vi "HMI.vi"() -> ()   [LabVIEW 2019, in "HMI Class 3.lvclass"]
uses:
  HMI Class 3.lvclass
  Class 2.lvclass
  Datos Out.vi
  Datos In.vi
panel:
  in  "MODO PRODUCCION":bool
  out "mensajes a usuario":string
  in  "PARO DE E":bool
  in  "Test":bool
  out "Numeric":dbl
  in  "MODO MANUAL":bool
  in  "stop":bool
  in  "INICIO":bool
  out "FALLA PRESENTE":bool
  out "MAQUINA EN ORIGEN":bool
  in  "RESET":bool
  in  "Tab Control":enum32{"0", "1", "2", "3", "4"}(tab)
  in  "MOVER A ORIGEN":bool
  in  "Nombre":string
  in  "Clave":string
  in  "ENTER":bool
  out "?":string
  out "PIEZAS YIELD":string
  out "PIEZAS MALAS":string
  out "LOTE ACTUAL":string
  out "JOB":string
  out "MODELO":string
  out "PIEZA 2":bool
  out "PIEZA":bool
  out "LIMITE MINIMO":dbl min=0.0 max=9999.0
  out "LIMITE MAXIMO":dbl min=0.0 max=9999.0
  out "LIMITE MINIMO":dbl min=0.0 max=9999.0
  out "LIMITE MAXIMO":dbl min=0.0 max=9999.0
  out "ESTADO DE PIEZA TENSION":string
  out "ESTADO DE PIEZA GAP":string
  out "VALOR DE DISTANCIA":dbl
  out "SIN CAMBIOS":bool
  out "PIEZAS BUENAS":string
  out "CON CAMBIOS":bool
  out "VALOR DE TENSIÓN":dbl
  out "SMAC SEGURO":bool
  out "PIEZA EN NIDO":bool
  in  "MANUAL":bool
  out "SMAC MUESTRA":bool
  out "SMAC APROX":bool
  in  "SMAC AVANZANDO":bool
  in  "SMAC RETORNANDO":bool
  in  "CILINDRO 2":bool
  in  "CILINDRO 1":bool
  out "SMAC AV. SEGURO":bool
  out "SMAC HOME":bool
  out "BIMANUAL 2":bool
  out "BIMANUAL 1":bool
  out "AVANCE CILINDRO 2":bool
  out "HOME CILINDRO 2":bool
  out "AVANCE CILINDRO 1":bool
  out "HOME CILINDRO 1":bool
  out "PIEZA":bool
  in  "LIMITE MINIMO":dbl min=0.0 max=9999.0
  in  "LIMITE MAXIMO 4":dbl min=0.0 max=9999.0
  out "ESTADO DE PIEZA GAP":string
  out "VALOR DE DISTANCIA":dbl
  in  "EST 2":bool
  out "PIEZA":bool
  in  "LIMITE MINIMO":dbl min=0.0 max=9999.0
  in  "LIMITE MAXIMO":dbl min=0.0 max=9999.0
  out "ESTADO DE PIEZA TENSION":string
  out "VALOR DE TENSIÓN":dbl
  in  "EST 1":bool
  out "SIN CAMBIOS":bool
  out "CON CAMBIOS":bool
  in  "EST 3":bool
  in  "MODO INGENIERIA":bool
  in  "MODO DE OPERACION":bool
  # "MENÚ PRINCIPAL"
  # "MODO DE OPERACIÓN"
  # "ESTACION 1\n PRUEBA TENSIÓN"
  # "ESTACION 2\n PRUEBA GAP"
  # "ESTACION 3\n PRUEBA TRIP-GAP"
  # "CONTINUAIDAD EN CONTACTOS"
  # "PRODUCCIÓN"
  # "SENSORES"
  # "CILINDROS"
  # "SEGURIDAD"
  # "ESTADO DEL SMAC"
  # "SMAC"
  # "ENTRADAS   MODO MANUAL    SALIDAS"
  # "SELECCION MODELO \nDE PIEZA"
  # "AGREGAR MODELO"
  # "ESTACION 1\n PRUEBA TENSIÓN"
  # "ESTACION 2\n PRUEBA GAP"
  # "ESTACION 3\n PRUEBA TRIP-GAP"
  # "CONTINUAIDAD EN CONTACTOS"
  # "MODO INGENIERIA\nCONFIGURACION DE PARAMETROS"
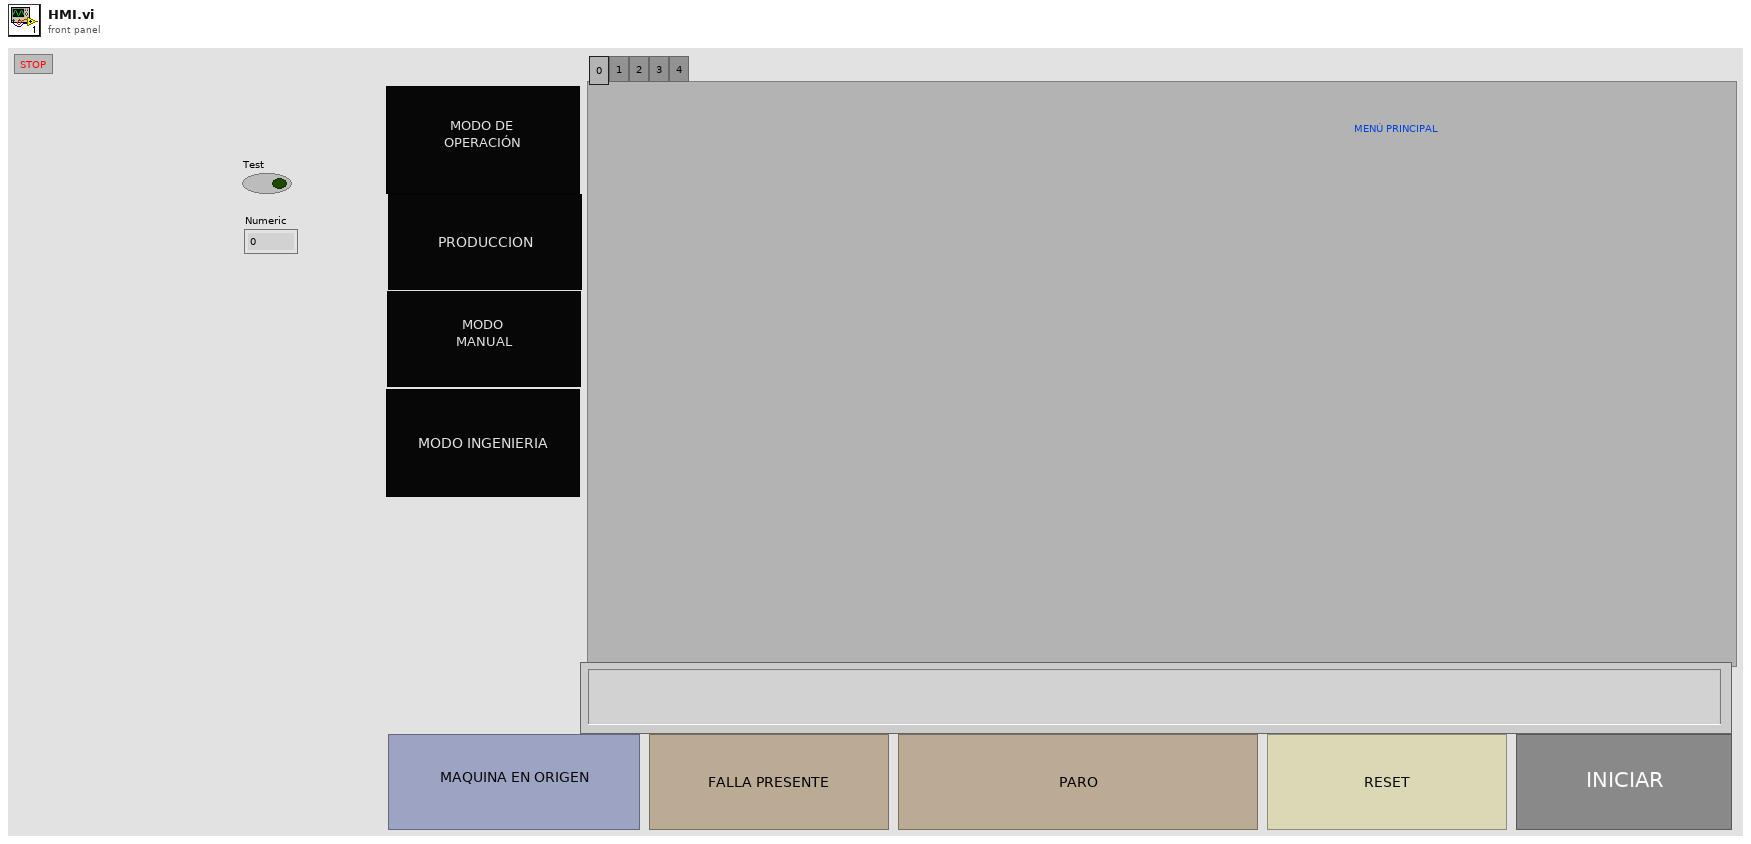
[diagram p1: front panel]
types:
  T1 = enum8{"Enabled", "Disabled", "Disabled and Grayed Out"}
  T2 = cluster{"Test":bool, "CILINDRO _1":bool, "CILINDRO _2":bool, "SMAC_RETORNANDO":bool, "SMAC_AVANZANDO":bool, "MANUAL":bool, "EST_1":bool, "EST_2":bool, "EST_3":bool, "MOVER A ORIGEN":bool, "RESET":bool, "PARO":bool, "INICIO":bool, "DATA_CONTROL":cluster{"ESTACION_1":cluster{"ACEPTADA":bool, "MAXIMO":dbl, "MINIMO":dbl, "LECTURA":dbl}, "ESTACION_2":cluster{"ACEPTADA":bool, "MAXIMO":dbl, "MINIMO":dbl, "LECTURA":dbl}, "ESTACION_3":cluster{"ACEPTADA":bool, "MAXIMO":dbl, "MINIMO":dbl, "LECTURA":dbl}}, "INGENIERIA O PROCESO":bool}
  T3 = cluster{"SALIDAS.CILINDRO 1":bool, "SALIDAS.CILINDRO 2":bool, "SALIDAS.SEMAC RETORNANDO":bool, "SALIDAS.SAMAC AVANZANDO":bool, "Auto(off)/Manual(on)":bool, "HOME_CILINDRO_1":bool, "HOME_CILINDRO_2":bool, "AVANCE_CILINDRO_1":bool, "AVANCE_CILINDRO_2":bool, "PIEZA_EN_NIDO":bool, "BIMANUAL 2":bool, "BIMANUAL1":bool, "SIN CAMBIOS":bool, "CON  CAMBIOS":bool, "TESTER":bool, "MAQUINA EN ORIGEN":bool, "FALLA PRESENTE":bool}
  T4 = cluster{"Numeric":dbl, "VALOR DE DISTANCIA":dbl, "VALOR DE TENSION":dbl}
  T5 = cluster{"DATO GAP":string, "DATO TENSION":string, "mensajes usuario":string}
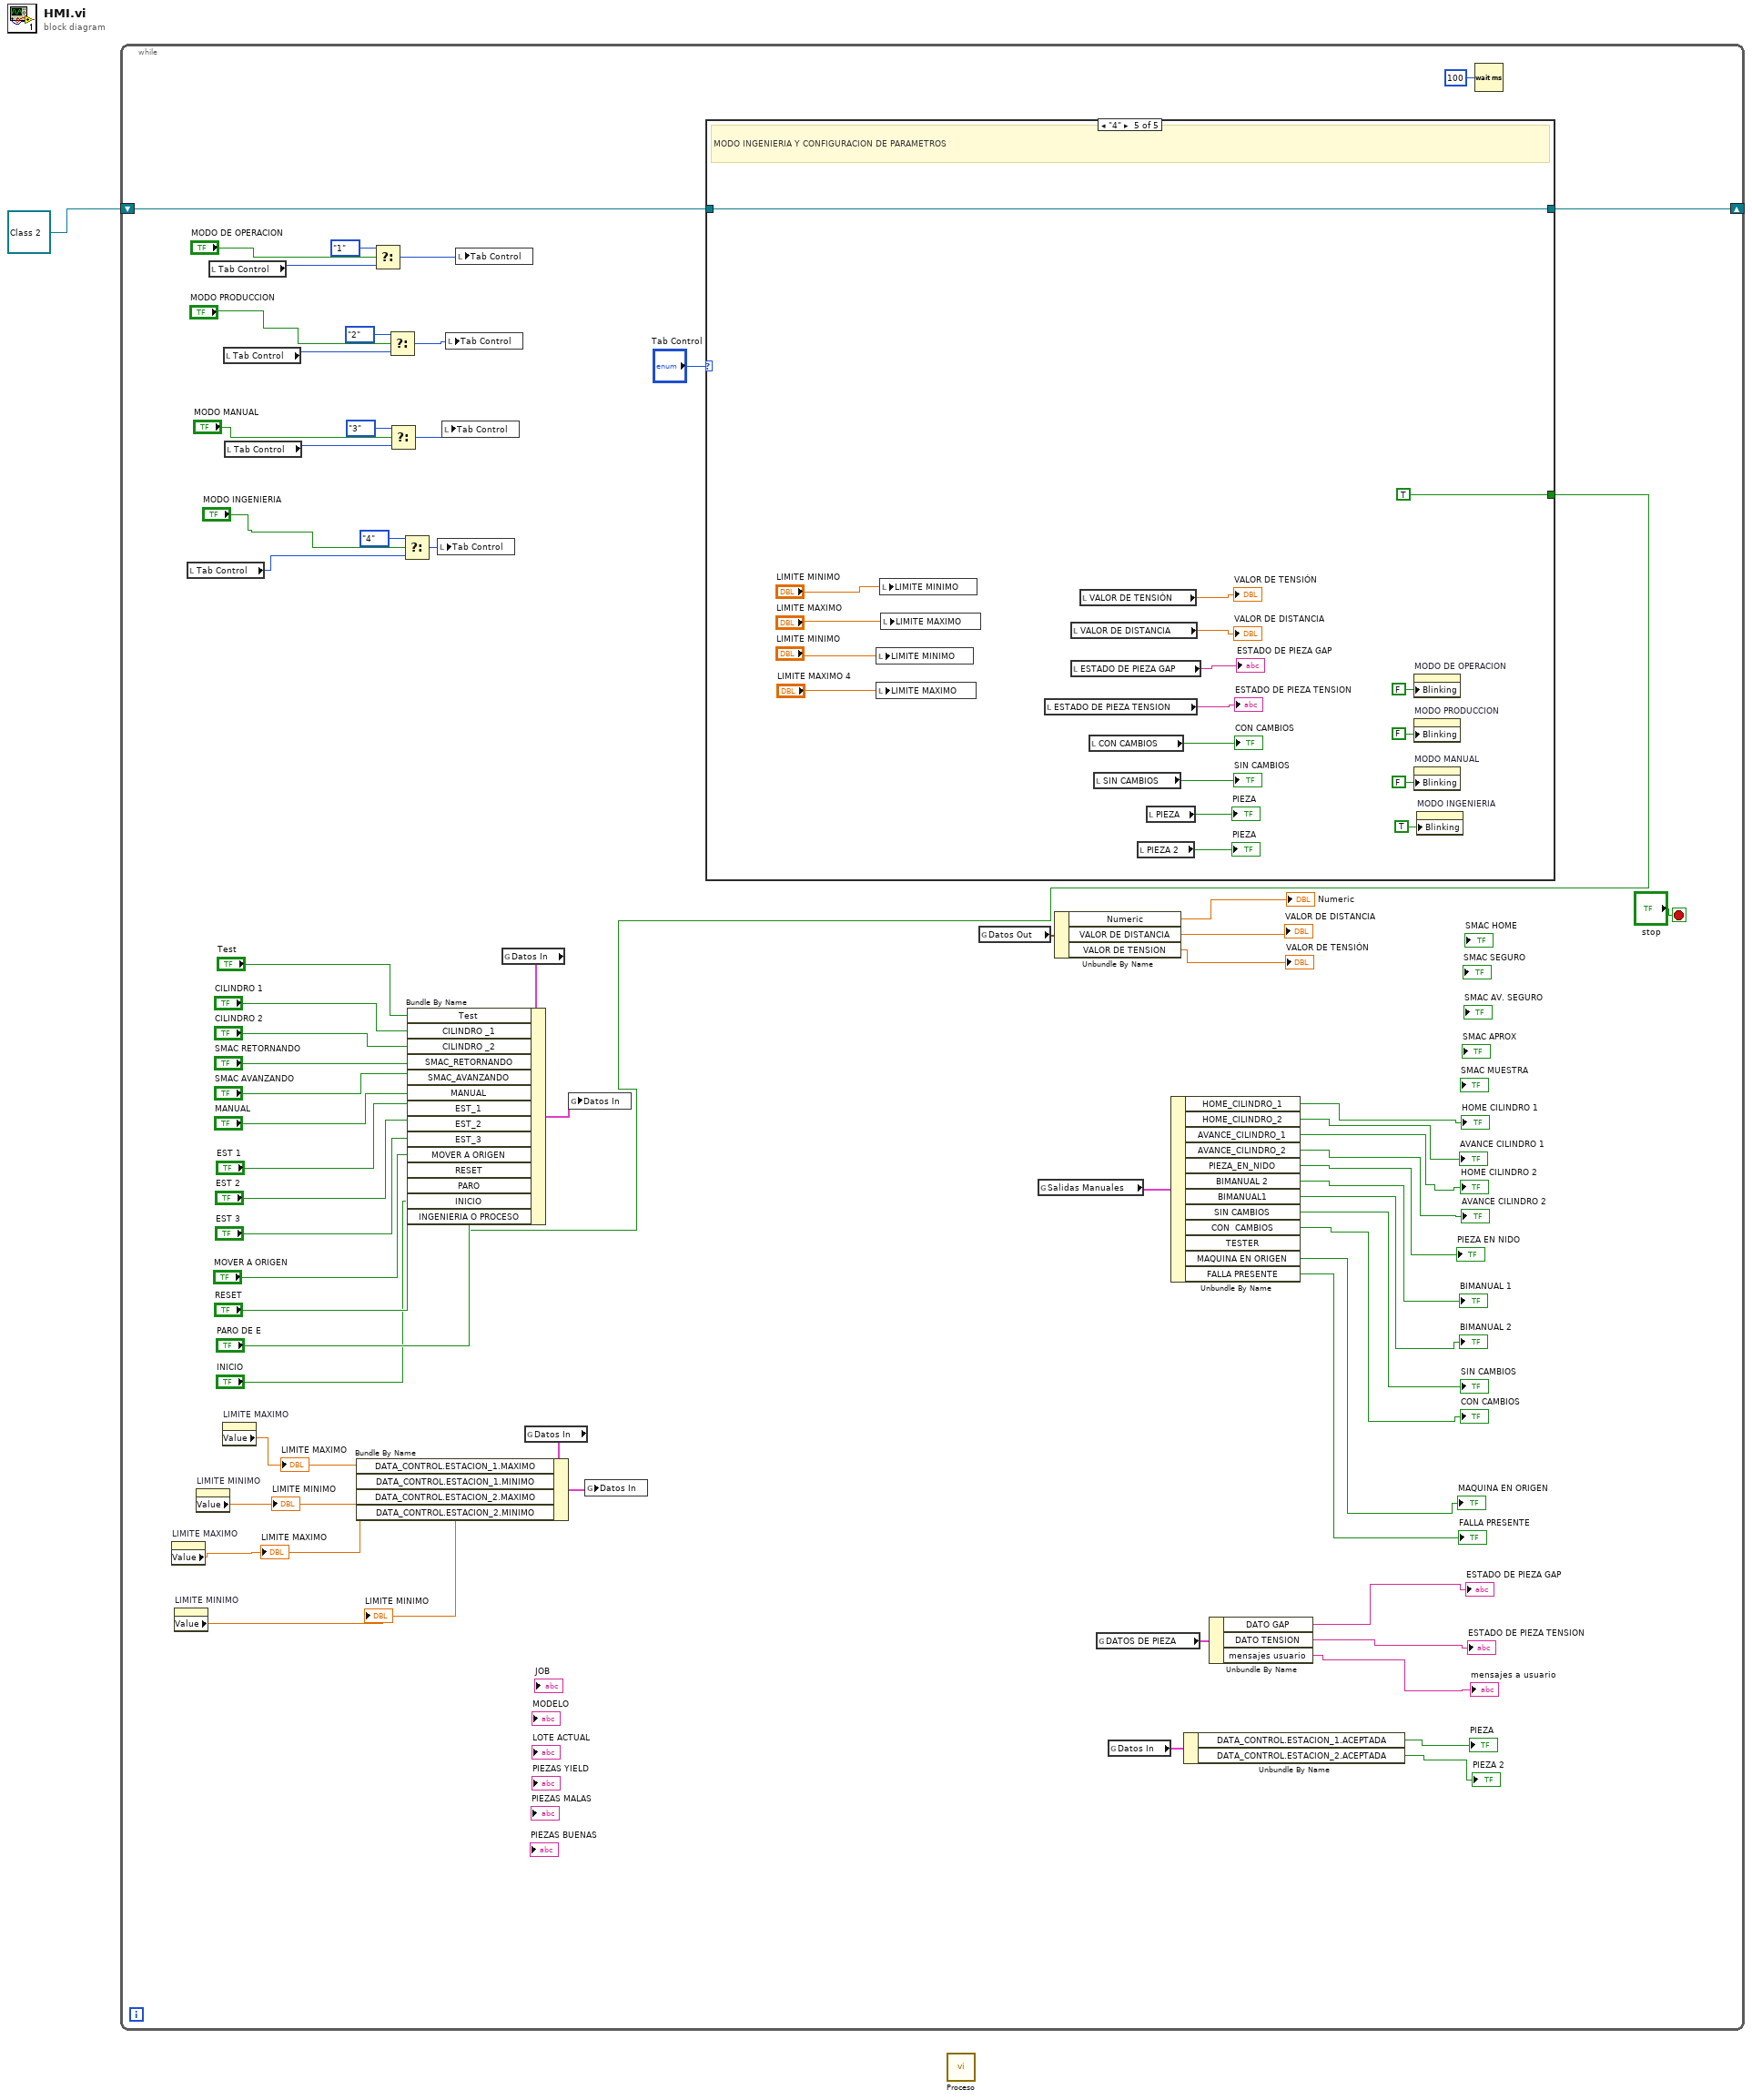
[diagram p0: block diagram]
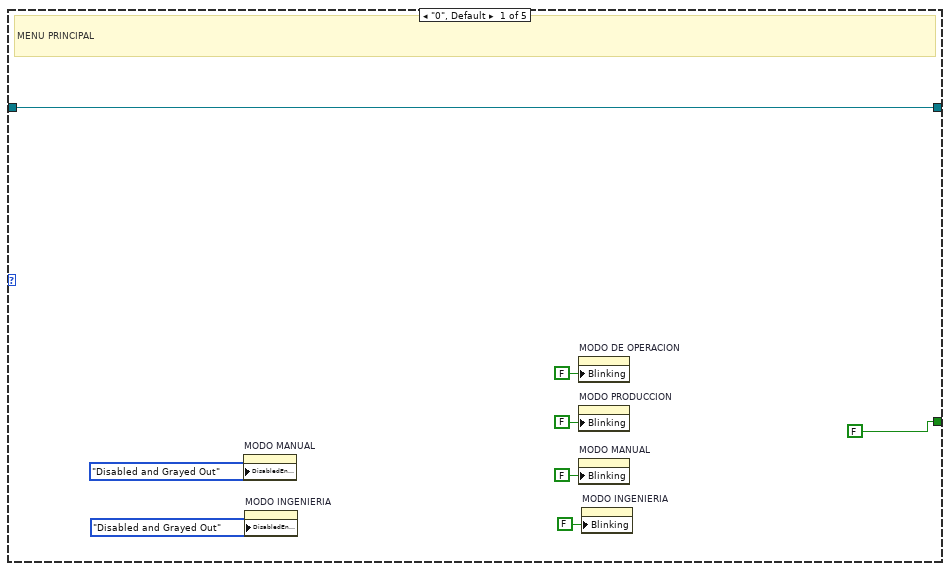
[diagram p2: hidden frame]
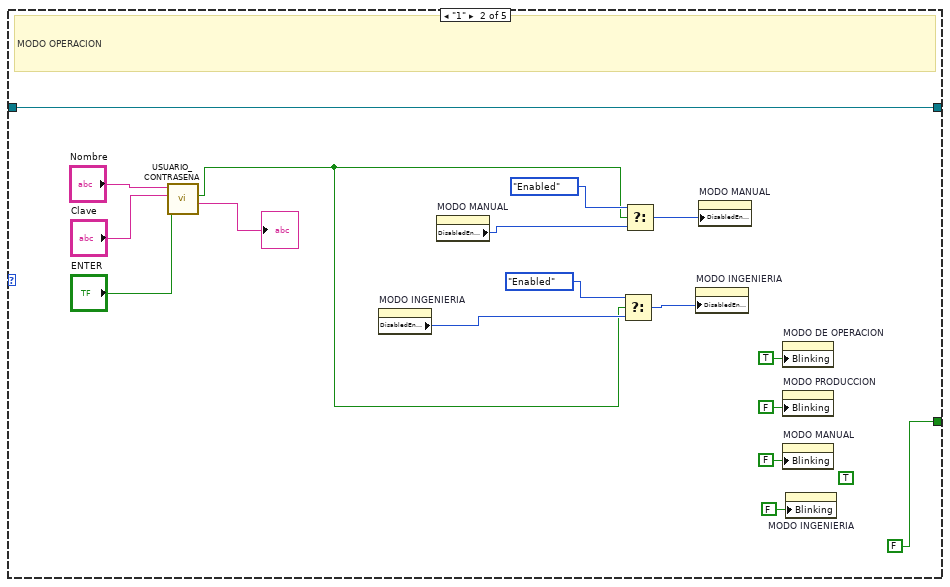
[diagram p3: hidden frame]
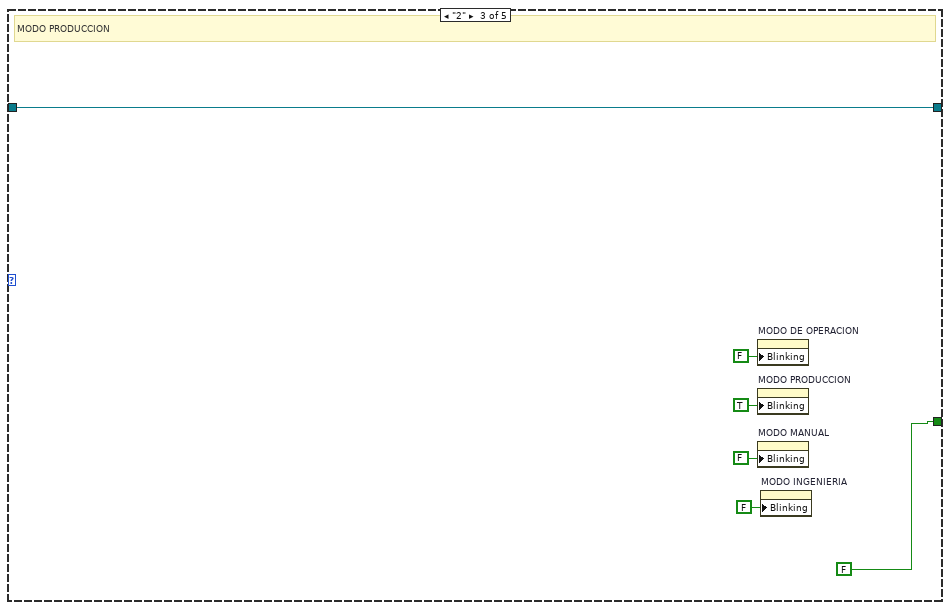
[diagram p4: hidden frame]
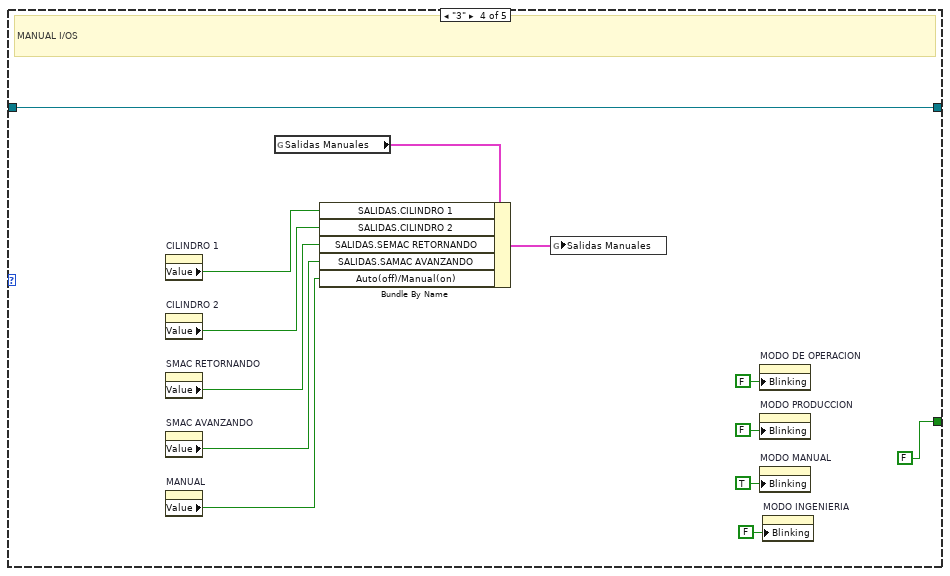
[diagram p5: hidden frame]
diagram:
  n1 = while {
    shift-right: [w64] -> _
    shift-left: refnum<class "Class 2.lvclass"> refnum ("Class 2.lvclass") -> [w65]
    stop <- "stop" stop-if-true
    n2 = property on="LIMITE MAXIMO" class="DigNum (strict)"() -> ("Value"=w4:dbl)  [unwired: 2 in, 2 out]
    "LIMITE MAXIMO" <- w4
    n3 = property on="LIMITE MINIMO" class="DigNum (strict)"() -> ("Value"=w5:dbl)  [unwired: 2 in, 2 out]
    "LIMITE MINIMO" <- w5
    n4 = local read "Tab Control"() -> (w19:enum32{"0", "1", "2", "3", "4"})
    n5 = property on="LIMITE MINIMO" class="DigNum (strict)"() -> ("Value"=w6:dbl)  [unwired: 2 in, 2 out]
    "LIMITE MINIMO" <- w6
    n6 = local read "Tab Control"() -> (w59:enum32{"0", "1", "2", "3", "4"})
    n7 = property on="LIMITE MAXIMO" class="DigNum (strict)"() -> ("Value"=w7:dbl)  [unwired: 2 in, 2 out]
    "LIMITE MAXIMO" <- w7
    n8 = local read "Tab Control"() -> (w11:enum32{"0", "1", "2", "3", "4"})
    n9 = local read "Tab Control"() -> (w15:enum32{"0", "1", "2", "3", "4"})
    n10 = Select(t=enum32{"0", "1", "2", "3", "4", "5", "6", "7"}."1", s="MODO DE OPERACION", f=w59) -> (s? t:f=w57:enum32{"0", "1", "2", "3", "4", "5", "6", "7"})
    n11 = Select(t=enum32{"0", "1", "2", "3", "4", "5", "6", "7"}."2", s="MODO PRODUCCION", f=w11) -> (s? t:f=w10:enum32{"0", "1", "2", "3", "4", "5", "6", "7"})
    n12 = Select(t=enum32{"0", "1", "2", "3", "4", "5", "6", "7"}."3", s="MODO MANUAL", f=w15) -> (s? t:f=w13:enum32{"0", "1", "2", "3", "4", "5", "6", "7"})
    n13 = Select(t=enum32{"0", "1", "2", "3", "4", "5", "6", "7"}."4", s="MODO INGENIERIA", f=w19) -> (s? t:f=w17:enum32{"0", "1", "2", "3", "4", "5", "6", "7"})
    n14 = local write "Tab Control"(w17) -> ()
    n15 = local write "Tab Control"(w13) -> ()
    n16 = local write "Tab Control"(w10) -> ()
    n17 = local write "Tab Control"(w57) -> ()
    n18 = global read "Datos In.vi" "Datos In"() -> (w31:T2)
    n19 = global read "Datos In.vi" "Datos In"() -> (w24:T2)
    n20 = Bundle By Name(cluster=w24, "DATA_CONTROL.ESTACION_1.MAXIMO"=w7, "DATA_CONTROL.ESTACION_1.MINIMO"=w6, "DATA_CONTROL.ESTACION_2.MAXIMO"=w4, "DATA_CONTROL.ESTACION_2.MINIMO"=w5) -> (w23:T2)
    n21 = global write "Datos In.vi" "Datos In"(w23) -> ()
    n22 = case shown="\"4\"" "Tab Control" {
      tunnel: w65 -> [w75 w92 w98 w111 w129]
      tunnel: [w75 w92 w98 w111 w129] -> w64
      tunnel: [FALSE FALSE FALSE FALSE TRUE] -> w2
      frame "0", Default {
        # "MENU PRINCIPAL"
        n23 = property on="MODO MANUAL" class="Bool (strict)"("DisabledEnum"=T1."Disabled and Grayed Out" ("Disabled")) -> ()  [unwired: 2 in, 2 out]
        n24 = property on="MODO INGENIERIA" class="Bool (strict)"("DisabledEnum"=T1."Disabled and Grayed Out" ("Disabled")) -> ()  [unwired: 2 in, 2 out]
        n25 = property on="MODO DE OPERACION" class="Bool (strict)"("Blinking"=FALSE) -> ()  [unwired: 2 in, 2 out]
        n26 = property on="MODO PRODUCCION" class="Bool (strict)"("Blinking"=FALSE) -> ()  [unwired: 2 in, 2 out]
        n27 = property on="MODO MANUAL" class="Bool (strict)"("Blinking"=FALSE) -> ()  [unwired: 2 in, 2 out]
        n28 = property on="MODO INGENIERIA" class="Bool (strict)"("Blinking"=FALSE) -> ()  [unwired: 2 in, 2 out]
      }
      frame "1" {
        (unwired) TRUE
        # "MODO OPERACION"
        n29 = call "USUARIO_CONTRASENA.vi"("INGRESAR (ENTER)"="ENTER", "Clave"="Clave", "Nombre"="Nombre") -> ("String 2"=→"?":string, "ACCESO"=w77:bool)  [unwired: 7 in]
        n30 = property on="MODO INGENIERIA" class="Bool (strict)"() -> ("DisabledEnum"=w86:T1)  [unwired: 2 in, 2 out]
        n31 = property on="MODO MANUAL" class="Bool (strict)"() -> ("DisabledEnum"=w87:T1)  [unwired: 2 in, 2 out]
        n32 = Select(t=T1."Enabled" ("Disabled"), s=w77, f=w86) -> (s? t:f=w90:T1)
        n33 = Select(t=T1."Enabled" ("Disabled"), s=w77, f=w87) -> (s? t:f=w91:T1)
        n34 = property on="MODO INGENIERIA" class="Bool (strict)"("DisabledEnum"=w90) -> ()  [unwired: 2 in, 2 out]
        n35 = property on="MODO MANUAL" class="Bool (strict)"("DisabledEnum"=w91) -> ()  [unwired: 2 in, 2 out]
        n36 = property on="MODO DE OPERACION" class="Bool (strict)"("Blinking"=TRUE) -> ()  [unwired: 2 in, 2 out]
        n37 = property on="MODO PRODUCCION" class="Bool (strict)"("Blinking"=FALSE) -> ()  [unwired: 2 in, 2 out]
        n38 = property on="MODO MANUAL" class="Bool (strict)"("Blinking"=FALSE) -> ()  [unwired: 2 in, 2 out]
        n39 = property on="MODO INGENIERIA" class="Bool (strict)"("Blinking"=FALSE) -> ()  [unwired: 2 in, 2 out]
      }
      frame "2" {
        # "MODO PRODUCCION"
        n40 = property on="MODO DE OPERACION" class="Bool (strict)"("Blinking"=FALSE) -> ()  [unwired: 2 in, 2 out]
        n41 = property on="MODO PRODUCCION" class="Bool (strict)"("Blinking"=TRUE) -> ()  [unwired: 2 in, 2 out]
        n42 = property on="MODO MANUAL" class="Bool (strict)"("Blinking"=FALSE) -> ()  [unwired: 2 in, 2 out]
        n43 = property on="MODO INGENIERIA" class="Bool (strict)"("Blinking"=FALSE) -> ()  [unwired: 2 in, 2 out]
      }
      frame "3" {
        # "MANUAL I/OS"
        n44 = property on="CILINDRO 1" class="Bool (strict)"() -> ("Value"=w110:bool)  [unwired: 2 in, 2 out]
        n45 = property on="CILINDRO 2" class="Bool (strict)"() -> ("Value"=w109:bool)  [unwired: 2 in, 2 out]
        n46 = property on="SMAC RETORNANDO" class="Bool (strict)"() -> ("Value"=w108:bool)  [unwired: 2 in, 2 out]
        n47 = property on="SMAC AVANZANDO" class="Bool (strict)"() -> ("Value"=w107:bool)  [unwired: 2 in, 2 out]
        n48 = property on="MANUAL" class="Bool (strict)"() -> ("Value"=w106:bool)  [unwired: 2 in, 2 out]
        n49 = global read "Datos Out.vi" "Salidas Manuales"() -> (w105:T3)
        n50 = Bundle By Name(cluster=w105, "SALIDAS.CILINDRO 1"=w110, "SALIDAS.CILINDRO 2"=w109, "SALIDAS.SEMAC RETORNANDO"=w108, "SALIDAS.SAMAC AVANZANDO"=w107, "Auto(off)/Manual(on)"=w106) -> (w104:T3)
        n51 = global write "Datos Out.vi" "Salidas Manuales"(w104) -> ()
        n52 = property on="MODO DE OPERACION" class="Bool (strict)"("Blinking"=FALSE) -> ()  [unwired: 2 in, 2 out]
        n53 = property on="MODO PRODUCCION" class="Bool (strict)"("Blinking"=FALSE) -> ()  [unwired: 2 in, 2 out]
        n54 = property on="MODO MANUAL" class="Bool (strict)"("Blinking"=TRUE) -> ()  [unwired: 2 in, 2 out]
        n55 = property on="MODO INGENIERIA" class="Bool (strict)"("Blinking"=FALSE) -> ()  [unwired: 2 in, 2 out]
      }
      frame "4" {
        # "MODO INGENIERIA Y CONFIGURACION DE PARAMETROS"
        n56 = local write "LIMITE MINIMO"("LIMITE MINIMO") -> ()
        n57 = local write "LIMITE MAXIMO"("LIMITE MAXIMO 4") -> ()
        n58 = local write "LIMITE MINIMO"("LIMITE MINIMO") -> ()
        n59 = local write "LIMITE MAXIMO"("LIMITE MAXIMO") -> ()
        n60 = local read "ESTADO DE PIEZA TENSION"() -> (→"ESTADO DE PIEZA TENSION":string)
        n61 = local read "VALOR DE DISTANCIA"() -> (→"VALOR DE DISTANCIA":dbl)
        n62 = local read "ESTADO DE PIEZA GAP"() -> (→"ESTADO DE PIEZA GAP":string)
        n63 = local read "VALOR DE TENSIÓN"() -> (→"VALOR DE TENSIÓN":dbl)
        n64 = local read "CON CAMBIOS"() -> (→"CON CAMBIOS":bool)
        n65 = local read "SIN CAMBIOS"() -> (→"SIN CAMBIOS":bool)
        n66 = local read "PIEZA 2"() -> (→"PIEZA":bool)
        n67 = local read "PIEZA"() -> (→"PIEZA":bool)
        n68 = property on="MODO DE OPERACION" class="Bool (strict)"("Blinking"=FALSE) -> ()  [unwired: 2 in, 2 out]
        n69 = property on="MODO PRODUCCION" class="Bool (strict)"("Blinking"=FALSE) -> ()  [unwired: 2 in, 2 out]
        n70 = property on="MODO MANUAL" class="Bool (strict)"("Blinking"=FALSE) -> ()  [unwired: 2 in, 2 out]
        n71 = property on="MODO INGENIERIA" class="Bool (strict)"("Blinking"=TRUE) -> ()  [unwired: 2 in, 2 out]
      }
    }
    n72 = Bundle By Name(cluster=w31, "Test"="Test", "CILINDRO _1"="CILINDRO 1", "CILINDRO _2"="CILINDRO 2", "SMAC_RETORNANDO"="SMAC RETORNANDO", "SMAC_AVANZANDO"="SMAC AVANZANDO", "MANUAL"="MANUAL", "EST_1"="EST 1", "EST_2"="EST 2", "EST_3"="EST 3", "MOVER A ORIGEN"="MOVER A ORIGEN", "RESET"="RESET", "PARO"="PARO DE E", "INICIO"="INICIO", "INGENIERIA O PROCESO"=w2) -> (w30:T2)
    n73 = global write "Datos In.vi" "Datos In"(w30) -> ()
    n74 = global read "Datos Out.vi" "Datos Out"() -> (w62:T4)
    n75 = global read "Datos Out.vi" "Salidas Manuales"() -> (w45:T3)
    n76 = Unbundle By Name(w62) -> ("Numeric"=→"Numeric":dbl, "VALOR DE DISTANCIA"=→"VALOR DE DISTANCIA":dbl, "VALOR DE TENSION"=→"VALOR DE TENSIÓN":dbl)
    n77 = global read "Datos Out.vi" "DATOS DE PIEZA"() -> (w28:T5)
    n78 = global read "Datos In.vi" "Datos In"() -> (w22:T2)
    n79 = Unbundle By Name(w45) -> ("HOME_CILINDRO_1"=→"HOME CILINDRO 1":bool, "HOME_CILINDRO_2"=→"AVANCE CILINDRO 1":bool, "AVANCE_CILINDRO_1"=→"HOME CILINDRO 2":bool, "AVANCE_CILINDRO_2"=→"AVANCE CILINDRO 2":bool, "PIEZA_EN_NIDO"=→"PIEZA EN NIDO":bool, "BIMANUAL 2"=→"BIMANUAL 1":bool, "BIMANUAL1"=→"BIMANUAL 2":bool, "SIN CAMBIOS"=→"SIN CAMBIOS":bool, "CON  CAMBIOS"=→"CON CAMBIOS":bool, "MAQUINA EN ORIGEN"=→"MAQUINA EN ORIGEN":bool, "FALLA PRESENTE"=→"FALLA PRESENTE":bool)  [unwired: 1 out]
    n80 = Unbundle By Name(w22) -> ("DATA_CONTROL.ESTACION_1.ACEPTADA"=→"PIEZA":bool, "DATA_CONTROL.ESTACION_2.ACEPTADA"=→"PIEZA 2":bool)
    n81 = Unbundle By Name(w28) -> ("DATO GAP"=→"ESTADO DE PIEZA GAP":string, "DATO TENSION"=→"ESTADO DE PIEZA TENSION":string, "mensajes usuario"=→"mensajes a usuario":string)
    n82 = Wait (ms)(milliseconds to wait=u32 100) -> ()  [unwired: 1 out]
  }
  n83 = call "Proceso.vi"() -> ()  [unwired: 12 in]
